vi "alignLeft.vi"(6 "ignoreCaption&Labels":bool, 8 "error in (no error)":errorcluster, 11 "refs":refnum<vi>[](array[refnum])) -> (0 "error out":errorcluster, 3 "refs(dup)":refnum<vi>[](array[refnum]))   [LabVIEW 2023, in "TLC_Geometry.lvlib"]
doc: "Aligns all controls to the leftmost position among the input controls.\nThe minimum X coordinate is computed and applied to all controls."
uses:
  TLC_Geometry.lvlib
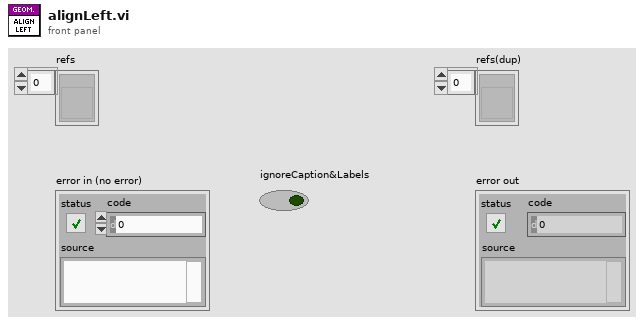
[diagram p1: front panel]
types:
  T1 = cluster{"left":i32, "top":i32, "right":i32, "bottom":i32}
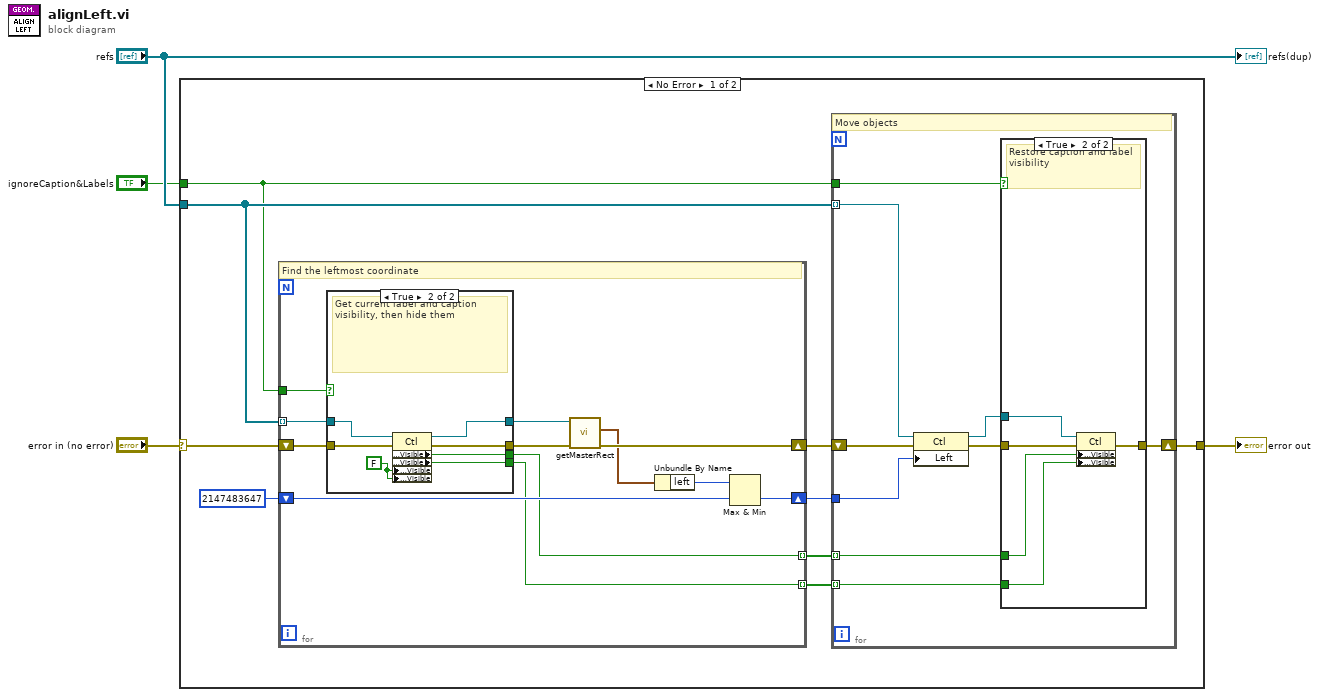
[diagram p0: block diagram]
diagram:
  n1 = case shown="No Error" "error in (no error)" {
    selector: "error in (no error)" -> [w13 w50]
    tunnel: [w10 w50] -> w4
    tunnel: "refs" -> [w11 _]
    tunnel: "ignoreCaption&Labels" -> [w7 _]
    frame No Error {
      n2 = for {
        tunnel: w11 -> [w35] mode=indexing
        shift-right: [w40] -> w9
        shift-left: w13 -> [w34]
        shift-right: [w29] -> w8
        shift-left: 2147483647 -> [w38]
        tunnel: w7 -> [w32]
        tunnel: [w31] -> w6 mode=indexing
        tunnel: [w30] -> w5 mode=indexing
        # "Find the leftmost coordinate"
        n3 = case shown="True" w32 {
          tunnel: [w42 w49] -> w36
          tunnel: w35 -> [w42 w48]
          tunnel: w34 -> [w41 w47]
          tunnel: [w41 w46] -> w33
          tunnel: [_ w45] -> w31
          tunnel: [_ w44] -> w30
          frame False {
            # "Do nothing"
          }
          frame True {
            w43 = FALSE ("Caption.Visible")
            # "Get current label and caption visibility, then hide them"
            n4 = property class="Ctl"(reference=w48, error in=w47, "Caption.Visible"=w43, "Label.Visible"=w43) -> (reference out=w49:refnum<vi>, error out=w46:errorcluster, "Caption.Visible"=w45:bool, "Label.Visible"=w44:bool)
          }
        }
        n5 = call "getMasterRect.vi"("error in (no error)"=w33, "ref"=w36) -> ("error out"=w40:errorcluster, "rect"=w37:T1)  [unwired: 7 in, 1 out]
        n6 = Unbundle By Name(w37) -> ("left"=w39:i32)
        n7 = Max & Min(x=w39, y=w38) -> (min(x,y)=w29:i32)  [unwired: 1 out]
      }
      n8 = for {
        tunnel: w11 -> [w22] mode=indexing
        shift-right: [w19] -> w10
        shift-left: w9 -> [w20]
        tunnel: w8 -> [w21]
        tunnel: w7 -> [w17]
        tunnel: w6 -> [w15] mode=indexing
        tunnel: w5 -> [w14] mode=indexing
        # "Move objects"
        n9 = property class="Ctl"(reference=w22, error in=w20, "Left"=w21) -> (reference out=w16:refnum<vi>, error out=w18:errorcluster)
        n10 = case shown="True" w17 {
          tunnel: w16 -> [_ w28]
          tunnel: w18 -> [w23 w27]
          tunnel: [w23 w26] -> w19
          tunnel: w15 -> [_ w25]
          tunnel: w14 -> [_ w24]
          frame False {
            # "Do nothing"
          }
          frame True {
            # "Restore caption and label visibility"
            n11 = property class="Ctl"(reference=w28, error in=w27, "Caption.Visible"=w25, "Label.Visible"=w24) -> (error out=w26:errorcluster)  [unwired: 1 out]
          }
        }
      }
    }
    frame Error {
    }
  }
  "error out" <- w4
  "refs(dup)" <- "refs"
